vi "IniToken SaveInfoToFile.vi"(8 "error in (no error)":errorcluster, 10 "Array":T2(array[cluster]), 11 "Path":path=path "D:/Dropbox/_workingOn/LabVIEW-Developing-QuickDrops/src/user.lib/_NEVSTOP/_LabVIEW.ini/test.iniToken") -> (0 "error out":errorcluster, 3 "string":string)   [LabVIEW 2015]
uses:
  Def-IniTokenCluster.ctl
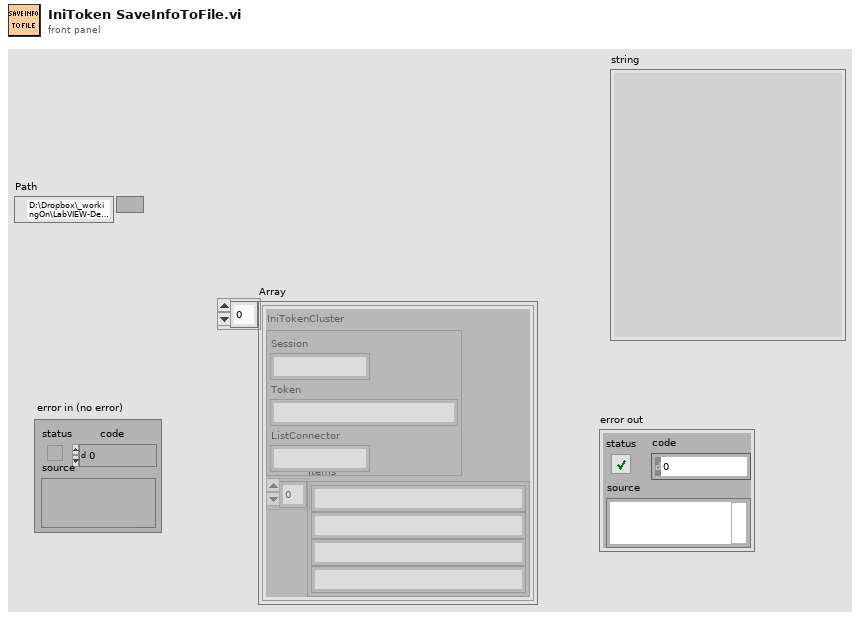
[diagram p1: front panel]
types:
  T1 = typedef "Def-IniTokenCluster.ctl" = cluster{"Session":string, "Token":string, "ListConnector":string}
  T2 = cluster{"IniTokenCluster":T1, "Items":string[]}[]
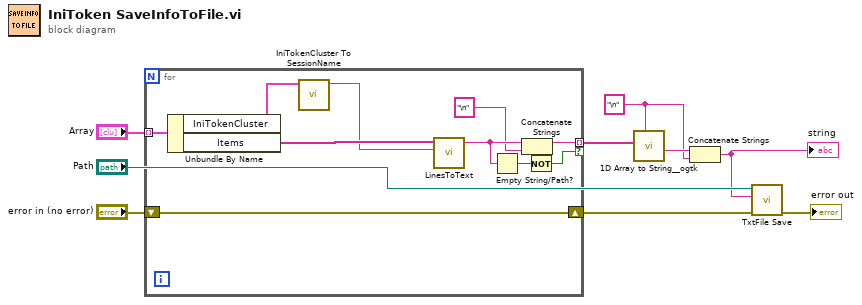
[diagram p0: block diagram]
diagram:
  w1 = "\n" ("delimiter (Tab)")
  n1 = for {
    shift-right: [w19] -> w3
    shift-left: "error in (no error)" -> [w19]
    tunnel: "Array" -> [w18] mode=indexing
    tunnel: [w10] -> w5 mode=indexing if=w13
    n2 = Unbundle By Name(w18) -> ("IniTokenCluster"=w17:T1, "Items"=w16:string[])
    n3 = call "IniTokenCluster To SessionName.vi"("IniTokenCluster"=w17) -> ("trimmed string"=w15:string)  [unwired: 10 in]
    n4 = call "LinesToText.vi"("Section(Empty)"=w15, "Lines"=w16) -> ("string"=w12:string)  [unwired: 8 in, 1 out]
    n5 = Empty String/Path?(string/path=w12) -> (empty?=w14:bool)
    n6 = Concatenate Strings(w12, "\n" ("delimiter (Tab)")) -> (w10:string)
    n7 = Not(x=w14) -> (.not. x?=w13:bool)
  }
  n8 = call <userlib>:"1D Array to String__ogtk.vi"("delimiter (Tab)"=w1, "Array of Strings"=w5) -> ("delimited string"=w4:string)  [unwired: 9 in]
  n9 = Concatenate Strings(w4, w1) -> (w2:string)
  "string" <- w2
  n10 = call "TxtFile Save.vi"("error in (no error)"=w3, "text"=w2, "Path"="Path") -> ("error out"=→"error out":errorcluster)  [unwired: 8 in]
